vi "ElevatorMaxHeightSendCmd.vi"(8 "error in (no error)":errorcluster) -> (0 "error out":errorcluster)   [LabVIEW 2023]
doc: "Currently unused Vi that sends a boolean command to the boolean receive called \"ElevMaxHeight\" (in ElevatorExecuteLogic.vi) to set Elevator to maximum height\nInputs:\n--error in\nOuputs:\n--error out"
uses:
  <vilib>/Rock Robotics/WPI/ThirdParty/JAS_Junk/TrajLib/Trajectory_Library.lvlib
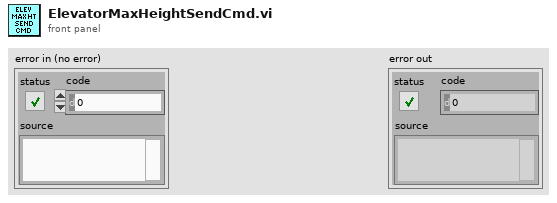
[diagram p1: front panel]
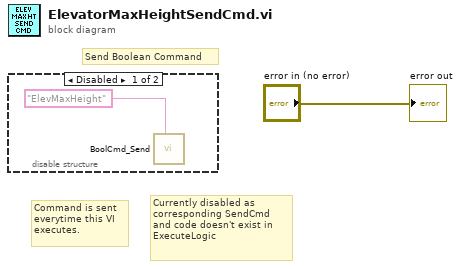
[diagram p0: block diagram]
diagram:
  # "Currently disabled as corresponding SendCmd and code doesn't exist in ExecuteLogic"
  # "Command is sent\neverytime this VI\nexecutes."
  # "Send Boolean Command"
  n1 = disable-structure shown="Disabled" {
    frame Disabled {
      n2 = call <vilib>:"BoolCmd_Send.vi"("Command Name"="ElevMaxHeight") -> ()  [unwired: 10 in, 1 out]
    }
    frame Enabled {
    }
  }
  "error out" <- "error in (no error)"
